vi "rmad to RegObs.vi"(7 "State":u16(ring)=1 items=["Init", "Write"], 10 "skredhendelse to regobs?":bool[](array[boolean]), 11 "Skredhendelser":T4(array[cluster]) {"Intensitet terskel 1" format="%.1f"; "Intensitet terskel 2" format="%.1f"; "Intensitet terskel 3" format="%.1f"; "Intensitet terskel 4" format="%.1f"; "Intensitet terskel 5" format="%.1f"}) -> (0 "error out":errorcluster, 1 "registration ID":string[](array[string]), 2 "registration in regObs":T1(array[cluster]) {"DestructiveSizeTID" items=["Ikke gitt"=0, "1-Harmløs"=1, "2-Små"=2, "3-Middels"=3, "4-Stort"=4, "5-Svært stort"=5, "Ukjent"=9]; "TerrainStartZoneTID" items=["Ikke gitt"=0, "Brattheng"=10, "Leområder"=20, "Nær rygg"=30, "I renne eller forsenkning"=40, "Svaberg"=50, "Skål"=60, "I skogen"=70, "Hogstfelt"=75, "Overalt i terrenget"=95, "Ukjent"=99]; "AvalancheTID" items=["Ikke gitt"=0, "Tørt løssnøskred"=12, "Vått løssnøskred"=11, "Tørt flakskred"=22, "Vått flakskred"=21, "Glideskred"=27, "Sørpeskred"=30, "Skavlfall"=40, "Ukjent"=99]; "AvalancheTriggerTID" items=["Ikke gitt"=0, "Naturlig utløst"=10, "Kunstig utløst"=20, "Ski eller skuter utløst"=21, "Ski eller skuter fjernutløst"=22, "Kunstig utløst testheng"=23, "Utløst med sprengstoff"=25, "Ukjent"=99]}, 3 "obs to regobs":T3, 5 "regobs from inifile":T2(array[cluster]) {"regobs_ObsLocation" items=["Ikke gitt"=0, "Lauvjuvet"=66553, "Sandneslia"=66555, "Lauvjuvet Demo"=47721, "Sandneslia Demo"=47724, "Lauvjuvet Test"=62943, "Sandneslia Test"=62942, "F46 Demo"=47760, "F46 test"=63942]; "regobs_AvalancheTriggerTID" items=["Ikke gitt"=0, "Naturlig utløst"=10, "Kunstig utløst"=20, "Ski eller skuter utløst"=21, "Ski eller skuter fjernutløst"=22, "Kunstig utløst testheng"=23, "Utløst med sprengstoff"=25, "Ukjent"=99]; "regobs_AvalancheTID" items=["Ikke gitt"=0, "Tørt løssnøskred"=12, "Vått løssnøskred"=11, "Tørt flakskred"=22, "Vått flakskred"=21, "Glideskred"=27, "Sørpeskred"=30, "Skavlfall"=40, "Ukjent"=99]; "regobs_TerrainStartZoneTID" items=["Ikke gitt"=0, "Brattheng"=10, "Leområder"=20, "Nær rygg"=30, "I renne eller forsenkning"=40, "Svaberg"=50, "Skål"=60, "I skogen"=70, "Hogstfelt"=75, "Overalt i terrenget"=95, "Ukjent"=99]}, 6 "baseurl":string)   [LabVIEW 2017]
uses:
  <vilib>/Utility/config.llb/Read Key (U32).vi
  <vilib>/Utility/config.llb/Read Key (String).vi
  <vilib>/Utility/config.llb/Read Key (Boolean).vi
  <vilib>/Utility/config.llb/Read Key (Double).vi
  <vilib>/Utility/config.llb/NI_LVConfig.lvlib
panel:
  out "value":bool
  out "obsLocation":cluster{"ObsLocationId":i32}
  out "DtObsTime":string
  out "num geofon noder":u32
  in  "initfile":string="rmad config svv.ini"
  in  "AvalancheObs":T3 {"DestructiveSizeTID" items=["Ikke gitt"=0, "1-Harmløs"=1, "2-Små"=2, "3-Middels"=3, "4-Stort"=4, "5-Svært stort"=5, "Ukjent"=9]; "AvalancheTriggerTID" items=["Ikke gitt"=0, "Naturlig utløst"=10, "Kunstig utløst"=20, "Ski eller skuter utløst"=21, "Ski eller skuter fjernutløst"=22, "Kunstig utløst testheng"=23, "Utløst med sprengstoff"=25, "Ukjent"=99]; "AvalancheTID" items=["Ikke gitt"=0, "Tørt løssnøskred"=12, "Vått løssnøskred"=11, "Tørt flakskred"=22, "Vått flakskred"=21, "Glideskred"=27, "Sørpeskred"=30, "Skavlfall"=40, "Ukjent"=99]; "TerrainStartZoneTID" items=["Ikke gitt"=0, "Brattheng"=10, "Leområder"=20, "Nær rygg"=30, "I renne eller forsenkning"=40, "Svaberg"=50, "Skål"=60, "I skogen"=70, "Hogstfelt"=75, "Overalt i terrenget"=95, "Ukjent"=99]}
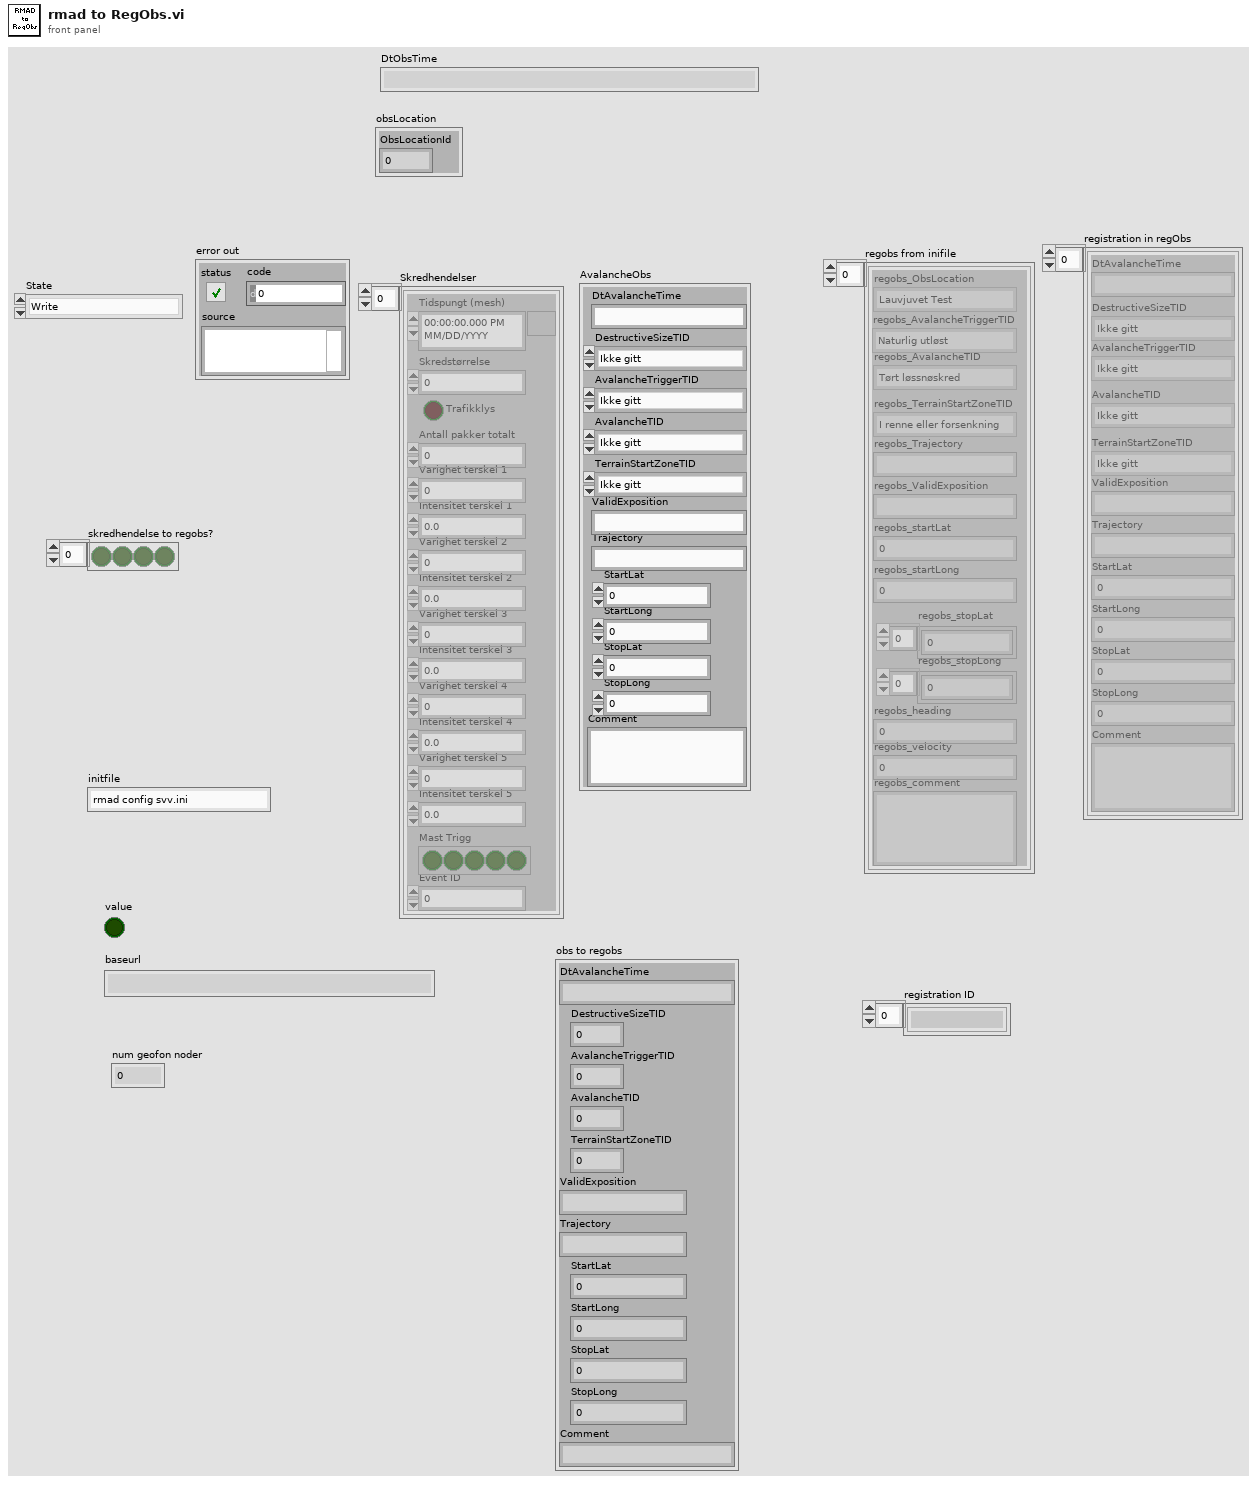
[diagram p1: front panel]
types:
  T1 = cluster{"DtAvalancheTime":string, "DestructiveSizeTID":i32, "AvalancheTriggerTID":i32, "AvalancheTID":i32, "TerrainStartZoneTID":i32, "ValidExposition":string, "Trajectory":string, "StartLat":dbl, "StartLong":dbl, "StopLat":dbl, "StopLong":dbl, "Comment":string}[]
  T2 = cluster{"regobs_ObsLocation":i32, "regobs_AvalancheTriggerTID":i32, "regobs_AvalancheTID":i32, "regobs_TerrainStartZoneTID":i32, "regobs_Trajectory":string, "regobs_ValidExposition":string, "regobs_startLat":dbl, "regobs_startLong":dbl, "regobs_stopLat":dbl[], "regobs_stopLong":dbl[], "regobs_heading":u32, "regobs_velocity":u32, "regobs_comment":string}[]
  T3 = cluster{"DtAvalancheTime":string, "DestructiveSizeTID":i32, "AvalancheTriggerTID":i32, "AvalancheTID":i32, "TerrainStartZoneTID":i32, "ValidExposition":string, "Trajectory":string, "StartLat":dbl, "StartLong":dbl, "StopLat":dbl, "StopLong":dbl, "Comment":string}
  T4 = cluster{"Tidspungt (mesh)":timestamp, "Skredstørrelse":u16, "Trafikklys":bool, "Antall pakker totalt":u16, "Varighet terskel 1":u16, "Intensitet terskel 1":dbl, "Varighet terskel 2":u16, "Intensitet terskel 2":dbl, "Varighet terskel 3":u16, "Intensitet terskel 3":dbl, "Varighet terskel 4":u16, "Intensitet terskel 4":dbl, "Varighet terskel 5":u16, "Intensitet terskel 5":dbl, "Mast Trigg":bool[], "Event ID":i32}[]
  T5 = cluster{"regobs_obsLocation":u32, "regobs_AvalancheTriggerTID":u32, "regobs_AvalancheTID":u32, "regobs_TerrainStartZoneTID":u32, "regobs_Trajectory":string, "regobs_ValidExposition":string, "regobs_startLat":dbl, "regobs_startLong":dbl, "regobs_stopLat":dbl[], "regobs_stopLong":dbl[], "regobs_heading":u32, "regobs_velocity":u32, "regobs_comment":string}
  T6 = typedef "NI_LVConfig.lvlib/Config Data RefNum.ctl" = refnum<k1>
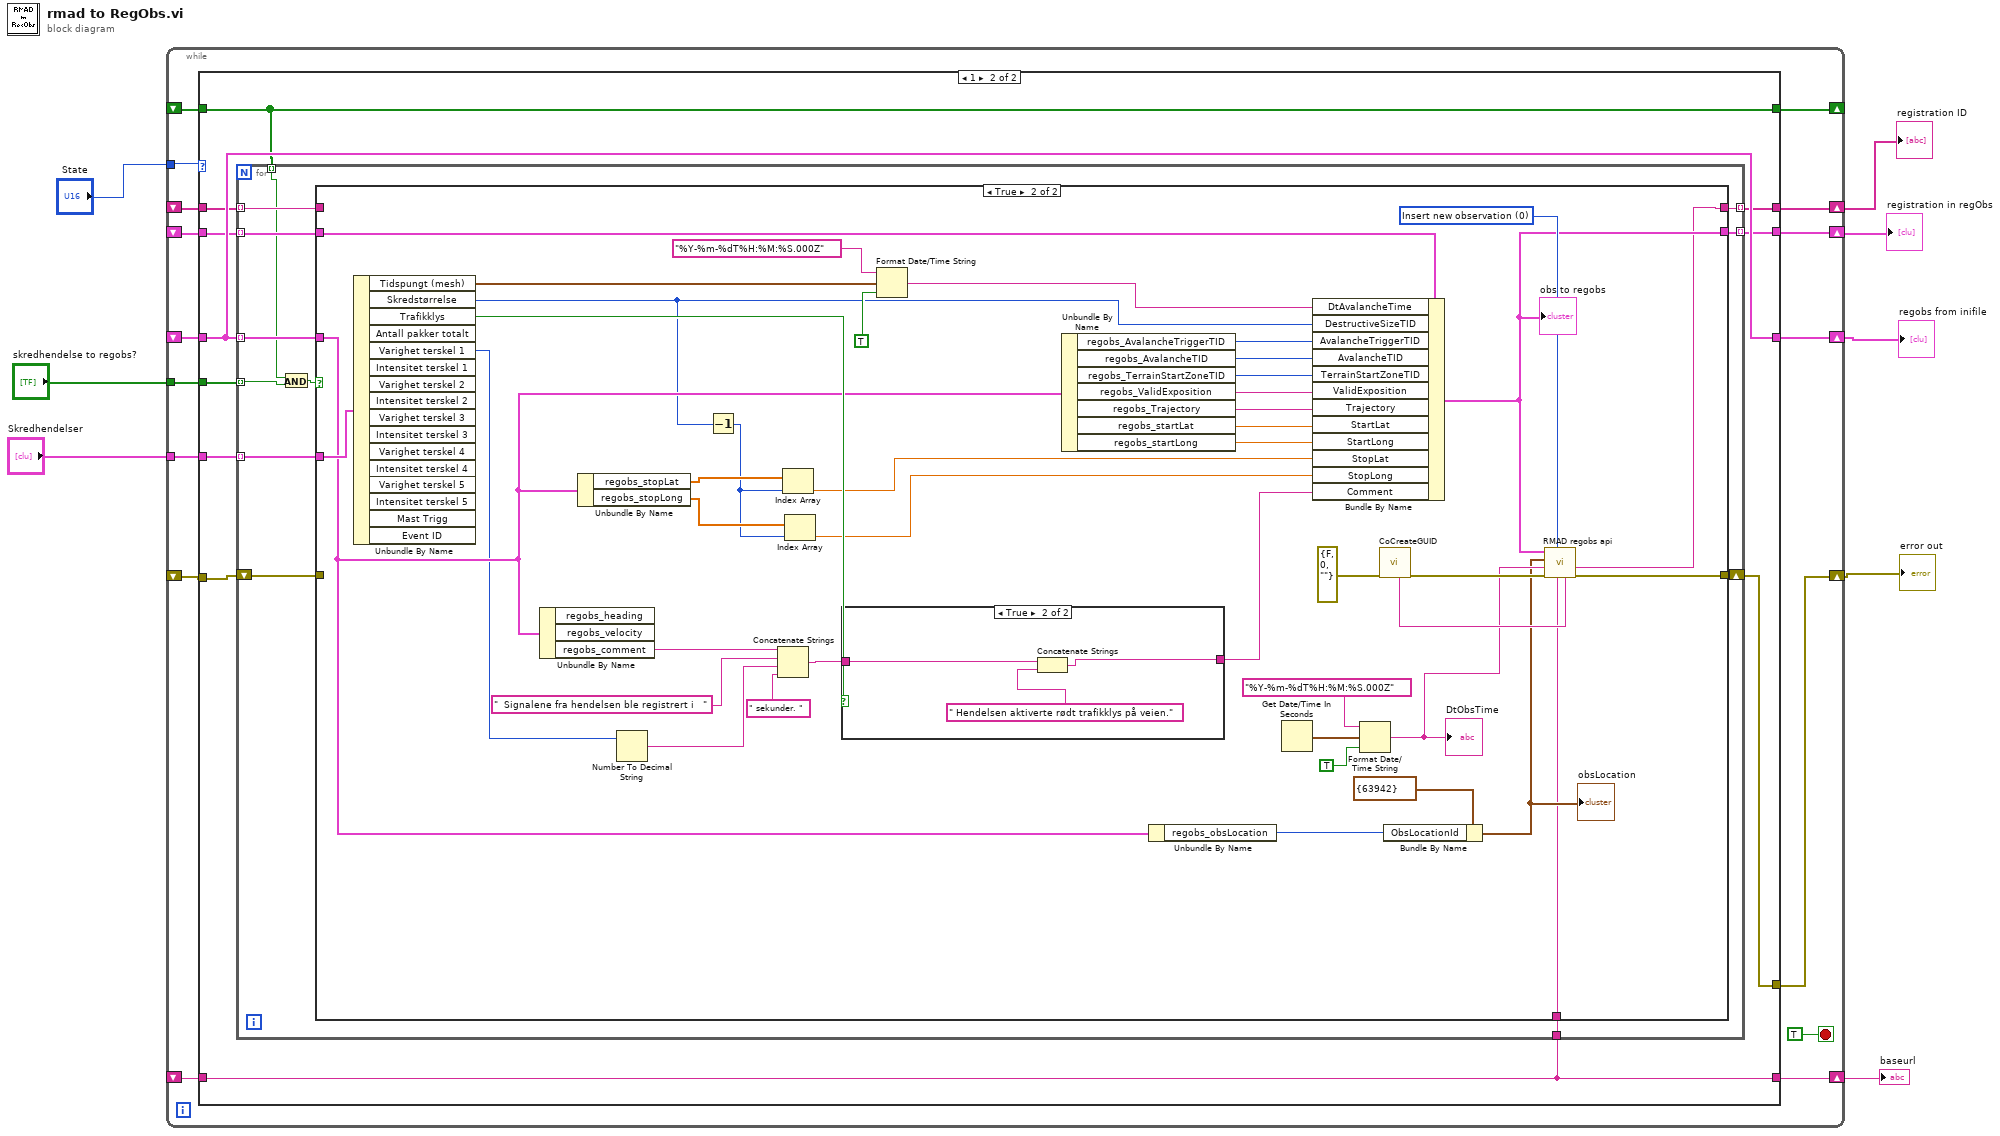
[diagram p0: block diagram]
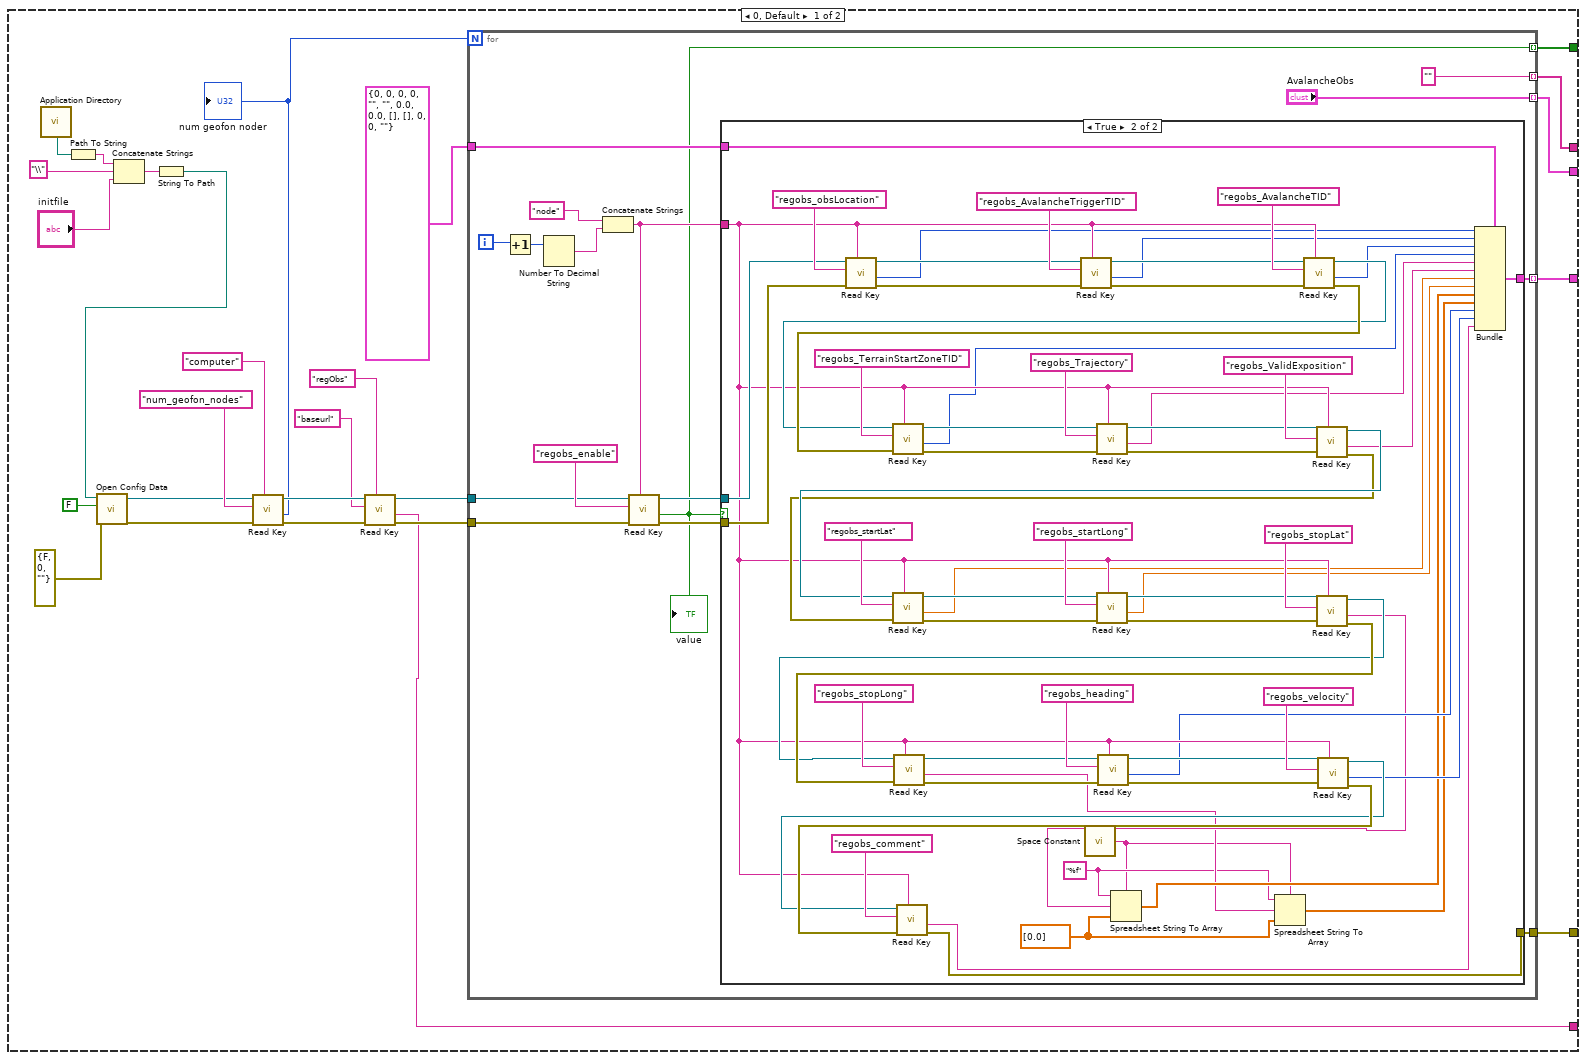
[diagram p2: hidden frame]
diagram:
  n1 = while {
    tunnel: "State" -> [w23]
    tunnel: "skredhendelse to regobs?" -> [w22]
    tunnel: "Skredhendelser" -> [w21]
    shift-right: [w20] -> w2
    shift-left: _ -> [w19]
    shift-right: [w18] -> w5
    shift-left: _ -> [w17]
    shift-right: [w16] -> w4
    shift-left: _ -> [w15]
    shift-right: [w14] -> w3
    shift-left: _ -> [w13]
    shift-right: [w12] -> w1
    shift-left: _ -> [w11]
    shift-right: [w10] -> _
    shift-left: _ -> [w9]
    stop <- TRUE stop-if-true
    n2 = case shown="1" w23 {
      tunnel: [w33 w140] -> w12
      tunnel: w11 -> [_ w139]
      tunnel: w22 -> [_ w138]
      tunnel: w21 -> [_ w137]
      tunnel: [w31 w136] -> w20
      tunnel: w19 -> [_ w136]
      tunnel: [w29 w135] -> w18
      tunnel: w17 -> [_ w134]
      tunnel: [w28 w133] -> w16
      tunnel: w15 -> [_ w132]
      tunnel: [w27 w131] -> w14
      tunnel: w13 -> [_ w131]
      tunnel: [w25 w130] -> w10
      tunnel: w9 -> [_ w130]
      frame 0, Default {
        n3 = call <vilib>:"Application Directory.vi"() -> ("Application Directory"=w50:path)
        n4 = Path To String(path=w50) -> (string=w49:string)
        n5 = Concatenate Strings(w49, "\\", "initfile") -> (w47:string)
        n6 = String To Path(string=w47) -> (path=w46:path)
        n7 = call <vilib>:"Open Config Data.vi"("error in (no error)"=errorcluster {"status"=FALSE, "code"=0, "source"=""}, "create file if necessary (T)"=FALSE, "configuration file path"=w46) -> ("error out"=w41:errorcluster, "refnum"=w40:T6)  [unwired: 6 in, 1 out]
        n8 = call-poly <vilib>:"Read Key.vi"("section"="computer", "error in (no error)"=w41, "key"="num_geofon_nodes", "refnum"=w40) -> ("error out"=w39:errorcluster, "value"=w32:u32, "refnum out"=w38:T6)  [unwired: 4 in, 1 out]
        "num geofon noder" <- w32
        n9 = call-poly <vilib>:"Read Key.vi"("section"="regObs", "error in (no error)"=w39, "key"="baseurl", "refnum"=w38) -> ("error out"=w34:errorcluster, "value"=w27:string, "refnum out"=w35:T6)  [unwired: 4 in, 1 out]
        n10 = for {
          N: w32 -> [_]
          tunnel: w34 -> [w60]
          tunnel: w35 -> [w61]
          tunnel: [w59] -> w33
          tunnel: [w55] -> w31 mode=indexing
          tunnel: T5 {"regobs_obsLocation"=0, "regobs_AvalancheTriggerTID"=0, "regobs_AvalancheTID"=0, "regobs_TerrainStartZoneTID"=0, "regobs_Trajectory"="", "regobs_ValidExposition"="", "regobs_startLat"=0.0, "regobs_startLong"=0.0, "regobs_stopLat"=[], "regobs_stopLong"=[], "regobs_heading"=0, "regobs_velocity"=0, "regobs_comment"=""} ("from inifile") -> [w54]
          tunnel: ["AvalancheObs"] -> w29 mode=indexing
          tunnel: ["" ("body insert 2")] -> w28 mode=indexing
          tunnel: [w51] -> w25 mode=indexing
          i -> [w63]
          n11 = Increment(x=w63) -> (x+1=w62:i32)
          n12 = Number To Decimal String(number=w62) -> (decimal integer string=w64:string)  [unwired: 1 in]
          n13 = Concatenate Strings("node" ("string"), w64) -> (w56:string)
          n14 = call-poly <vilib>:"Read Key.vi"("section"=w56, "error in (no error)"=w60, "key"="regobs_enable" ("section"), "refnum"=w61) -> ("error out"=w58:errorcluster, "value"=w51:bool, "refnum out"=w57:T6)  [unwired: 4 in, 1 out]
          "value" <- w51
          n15 = case shown="True" w51 {
            tunnel: [w68 w89] -> w59
            tunnel: w58 -> [w68 w128]
            tunnel: w57 -> [_ w127]
            tunnel: w56 -> [_ w90]
            tunnel: [w67 w77] -> w55
            tunnel: w54 -> [w67 w76]
            frame False {
            }
            frame True {
              w71 = dbl[] [0.0] ("array type (2D Dbl)")
              w70 = "%f" ("format string")
              n16 = call-poly <vilib>:"Read Key.vi"("section"=w90, "error in (no error)"=w128, "key"="regobs_obsLocation", "refnum"=w127) -> ("error out"=w123:errorcluster, "value"=w88:u32, "refnum out"=w124:T6)  [unwired: 4 in, 1 out]
              n17 = call-poly <vilib>:"Read Key.vi"("section"=w90, "error in (no error)"=w123, "key"="regobs_AvalancheTriggerTID", "refnum"=w124) -> ("error out"=w121:errorcluster, "value"=w87:u32, "refnum out"=w122:T6)  [unwired: 4 in, 1 out]
              n18 = call <vilib>:"Space Constant.vi"() -> ("String"=w69:string)
              n19 = call-poly <vilib>:"Read Key.vi"("section"=w90, "error in (no error)"=w121, "key"="regobs_AvalancheTID", "refnum"=w122) -> ("error out"=w117:errorcluster, "value"=w86:u32, "refnum out"=w116:T6)  [unwired: 4 in, 1 out]
              n20 = call-poly <vilib>:"Read Key.vi"("section"=w90, "error in (no error)"=w117, "key"="regobs_TerrainStartZoneTID", "refnum"=w116) -> ("error out"=w113:errorcluster, "value"=w85:u32, "refnum out"=w115:T6)  [unwired: 4 in, 1 out]
              n21 = call-poly <vilib>:"Read Key.vi"("section"=w90, "error in (no error)"=w113, "key"="regobs_Trajectory", "refnum"=w115) -> ("error out"=w112:errorcluster, "value"=w84:string, "refnum out"=w114:T6)  [unwired: 4 in, 1 out]
              n22 = call-poly <vilib>:"Read Key.vi"("section"=w90, "error in (no error)"=w112, "key"="regobs_ValidExposition", "refnum"=w114) -> ("error out"=w103:errorcluster, "value"=w83:string, "refnum out"=w104:T6)  [unwired: 4 in, 1 out]
              n23 = call-poly <vilib>:"Read Key.vi"("section"=w90, "error in (no error)"=w103, "key"="regobs_startLat", "refnum"=w104) -> ("error out"=w106:errorcluster, "value"=w82:dbl, "refnum out"=w108:T6)  [unwired: 4 in, 1 out]
              n24 = call-poly <vilib>:"Read Key.vi"("section"=w90, "error in (no error)"=w106, "key"="regobs_startLong", "refnum"=w108) -> ("error out"=w105:errorcluster, "value"=w81:dbl, "refnum out"=w107:T6)  [unwired: 4 in, 1 out]
              n25 = call-poly <vilib>:"Read Key.vi"("section"=w90, "error in (no error)"=w105, "key"="regobs_stopLat", "refnum"=w107) -> ("error out"=w95:errorcluster, "value"=w75:string, "refnum out"=w94:T6)  [unwired: 4 in, 1 out]
              n26 = call-poly <vilib>:"Read Key.vi"("section"=w90, "error in (no error)"=w95, "key"="regobs_stopLong", "refnum"=w94) -> ("error out"=w97:errorcluster, "value"=w73:string, "refnum out"=w99:T6)  [unwired: 4 in, 1 out]
              n27 = call-poly <vilib>:"Read Key.vi"("section"=w90, "error in (no error)"=w97, "key"="regobs_heading", "refnum"=w99) -> ("error out"=w96:errorcluster, "value"=w80:u32, "refnum out"=w98:T6)  [unwired: 4 in, 1 out]
              n28 = Spreadsheet String To Array(delimiter (Tab)=w69, format string=w70, spreadsheet string=w75, array type (2D Dbl)=w71) -> (array=w74:dbl[])
              n29 = Spreadsheet String To Array(delimiter (Tab)=w69, format string=w70, spreadsheet string=w73, array type (2D Dbl)=w71) -> (array=w72:dbl[])
              n30 = call-poly <vilib>:"Read Key.vi"("section"=w90, "error in (no error)"=w96, "key"="regobs_velocity", "refnum"=w98) -> ("error out"=w92:errorcluster, "value"=w79:u32, "refnum out"=w91:T6)  [unwired: 4 in, 1 out]
              n31 = call-poly <vilib>:"Read Key.vi"("section"=w90, "error in (no error)"=w92, "key"="regobs_comment", "refnum"=w91) -> ("error out"=w89:errorcluster, "value"=w78:string)  [unwired: 4 in, 2 out]
              n32 = Bundle(cluster=w76, "regobs_obsLocation"=w88, "regobs_AvalancheTriggerTID"=w87, "regobs_AvalancheTID"=w86, "regobs_TerrainStartZoneTID"=w85, "regobs_Trajectory"=w84, "regobs_ValidExposition"=w83, "regobs_startLat"=w82, "regobs_startLong"=w81, "regobs_stopLat"=w74, "regobs_stopLong"=w72, "regobs_heading"=w80, "regobs_velocity"=w79, "regobs_comment"=w78) -> (w77:T5)
            }
          }
        }
      }
      frame 1 {
        n33 = for {
          shift-right: [w152] -> w140
          shift-left: w139 -> [w151]
          tunnel: w138 -> [w142] mode=indexing
          tunnel: w137 -> [w150] mode=indexing
          tunnel: w136 -> [w149] mode=indexing
          tunnel: [w148] -> w135 mode=indexing
          tunnel: w134 -> [w147] mode=indexing
          tunnel: [w146] -> w133 mode=indexing
          tunnel: w132 -> [w145] mode=indexing
          tunnel: w131 -> [w144]
          tunnel: w130 -> [w141] mode=indexing
          n34 = And(x=w141, y=w142) -> (x .and. y?=w143:bool)
          n35 = case shown="True" w143 {
            tunnel: [w155 w198] -> w152
            tunnel: w151 -> [w155 _]
            tunnel: w150 -> [_ w194]
            tunnel: w149 -> [_ w170]
            tunnel: [w154 w173] -> w148
            tunnel: w147 -> [w154 w174]
            tunnel: [w153 w172] -> w146
            tunnel: w145 -> [w153 _]
            tunnel: w144 -> [_ w171]
            frame False {
            }
            frame True {
              w196 = u16 0 items=["Insert new observation", "Get observation"] ("State")
              n36 = Unbundle By Name(w194) -> ("Tidspungt (mesh)"=w187:timestamp, "Skredstørrelse"=w165:u16, "Trafikklys"=w177:bool, "Varighet terskel 1"=w163:u16)  [unwired: 12 out]
              n37 = Unbundle By Name(w170) -> ("regobs_comment"=w162:string)  [unwired: 2 out]
              n38 = Unbundle By Name(w170) -> ("regobs_stopLat"=w168:dbl[], "regobs_stopLong"=w169:dbl[])
              n39 = Number To Decimal String(number=w163) -> (decimal integer string=w160:string)  [unwired: 1 in]
              n40 = Decrement(x=w165) -> (x-1=w164:u16)
              n41 = Concatenate Strings(w162, "  Signalene fra hendelsen ble registrert i   " ("string"), w160, " sekunder. " ("string")) -> (w161:string)
              n42 = Index Array(array=w168, index=w164) -> (element=w167:dbl)
              n43 = Index Array(array=w169, index=w164) -> (element=w166:dbl)
              n44 = case shown="True" w177 {
                tunnel: [w199 w201] -> w157
                tunnel: w161 -> [w199 w202]
                frame False {
                }
                frame True {
                  n45 = Concatenate Strings(w202, " Hendelsen aktiverte rødt trafikklys på veien." ("string")) -> (w201:string)
                }
              }
              n46 = Format Date/Time String(time format string (%c)="%Y-%m-%dT%H:%M:%S.000Z", seconds (now)=w187, UTC format=TRUE) -> (date/time string=w186:string)
              n47 = Unbundle By Name(w170) -> ("regobs_AvalancheTriggerTID"=w184:u32, "regobs_AvalancheTID"=w183:u32, "regobs_TerrainStartZoneTID"=w182:u32, "regobs_ValidExposition"=w181:string, "regobs_Trajectory"=w180:string, "regobs_startLat"=w179:dbl, "regobs_startLong"=w178:dbl)
              n48 = Unbundle By Name(w170) -> ("regobs_obsLocation"=w185:u32)
              n49 = Get Date/Time In Seconds() -> (seconds since 1Jan1904=w193:timestamp)
              n50 = Bundle By Name(cluster=w174, "DtAvalancheTime"=w186, "DestructiveSizeTID"=w165, "AvalancheTriggerTID"=w184, "AvalancheTID"=w183, "TerrainStartZoneTID"=w182, "ValidExposition"=w181, "Trajectory"=w180, "StartLat"=w179, "StartLong"=w178, "StopLat"=w167, "StopLong"=w166, "Comment"=w157) -> (w173:T3)
              "obs to regobs" <- w173
              n51 = Format Date/Time String(time format string (%c)="%Y-%m-%dT%H:%M:%S.000Z", seconds (now)=w193, UTC format=TRUE) -> (date/time string=w191:string)
              "DtObsTime" <- w191
              n52 = call "CoCreateGUID.vi"("error in (no error)"=errorcluster {"status"=FALSE, "code"=0, "source"=""}) -> ("error out"=w197:errorcluster, "GUID string"=w195:string)  [unwired: 8 in, 1 out]
              n53 = Bundle By Name(cluster=cluster{"ObsLocationId":i32} {"ObsLocationId"=63942} ("ObsLocation"), "ObsLocationId"=w185) -> (w189:cluster{"ObsLocationId":i32})
              "obsLocation" <- w189
              n54 = call "RMAD regobs api.vi"("Id"=w195, "base url"=w171, "State"=w196, "error in (no error)"=w197, "DtObsTime"=w191, "ObsLocation"=w189, "AvalancheObs"=w173) -> ("error out"=w198:errorcluster, "body insert"=w172:string)  [unwired: 2 in, 1 out]
            }
          }
        }
      }
    }
  }
  "error out" <- w1
  "regobs from inifile" <- w2
  "registration in regObs" <- w5
  "registration ID" <- w4
  "baseurl" <- w3
